vi "Get SMO Port.vi"(8 "error in (no error)":errorcluster, 11 "Instrument.Framework-Template in":refnum<class "Instrument.Framework-Template.lvclass">) -> (0 "error out":errorcluster, 2 "Port":u16, 3 "Instrument.Framework-Template out":refnum<class "Instrument.Framework-Template.lvclass">)   [LabVIEW 2019, in "Instrument.Framework-Template.lvclass"]
uses:
  Instrument.Framework-Template.lvclass
  <userlib>/LevyLab/Instrument Framework/Instrument Types/SCPI/Instrument.SCPI.lvclass
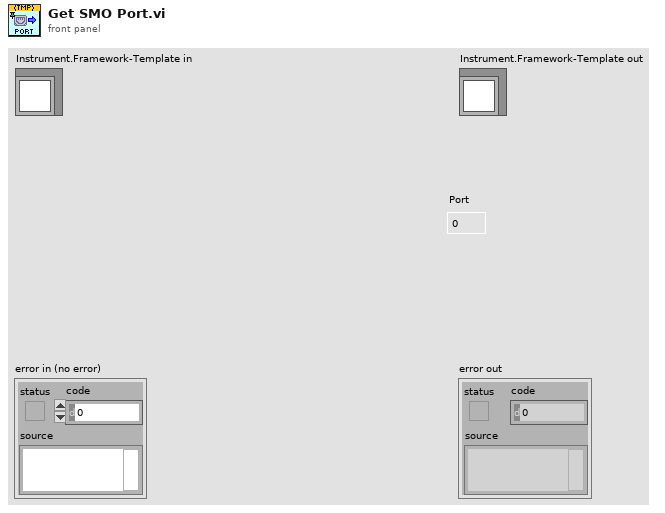
[diagram p1: front panel]
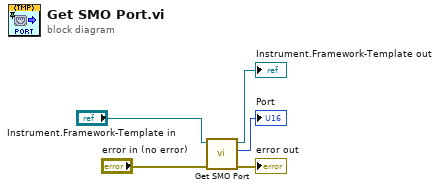
[diagram p0: block diagram]
diagram:
  n1 = call-parent "Get SMO Port.vi"("error in (no error)"="error in (no error)", "Instrument in"="Instrument.Framework-Template in") -> ("error out"=→"error out":errorcluster, "Port"=→"Port":u16, "Instrument out"=→"Instrument.Framework-Template out":refnum<class "Instrument.Framework-Template.lvclass">)  [unwired: 7 in]
